vi "Content.vi"(7 "Context":refnum<class "Context.lvclass">, 8 "Error In":errorcluster, 11 "Text In":refnum<class "Text.lvclass">) -> (0 "Error Out":errorcluster, 2 "Content":string, 3 "Text Out":refnum<class "Text.lvclass">)   [LabVIEW 2018, in "Toolkit.lvlib" / "Nodes.lvlib" / "Text.lvclass"]
uses:
  Text.lvclass
  Support/Context/Context.lvclass
  Text.lvclass/Text.ctl
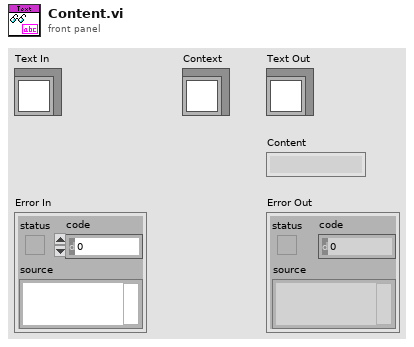
[diagram p1: front panel]
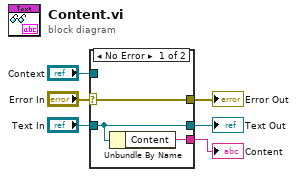
[diagram p0: block diagram]
diagram:
  n1 = case shown="No Error" "Error In" {
    selector: "Error In" -> [w9 w11]
    tunnel: [w9 w11] -> w5
    tunnel: "Text In" -> [w8 w10]
    tunnel: [w8 w10] -> w3
    tunnel: [w7 _] -> w2
    tunnel: "Context" -> [_ _]
    frame No Error {
      n2 = Unbundle By Name(w8) -> ("Content"=w7:string)
    }
    frame Error {
    }
  }
  "Error Out" <- w5
  "Text Out" <- w3
  "Content" <- w2
